vi "MP_Conver_HumanToMachine.vi"(6 "Vel_In (ft/s)":dbl, 7 "Pos_In (ft)":dbl, 8 "CPR":dbl, 9 "Diameter (ft)":dbl) -> (2 "Vel_Out (u/100ms)":dbl, 3 "Pos_Out (u)":dbl)   [LabVIEW 2017]
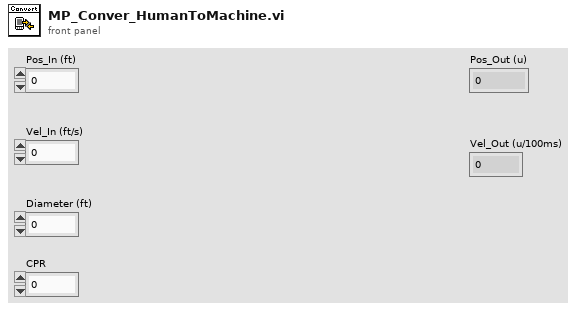
[diagram p1: front panel]
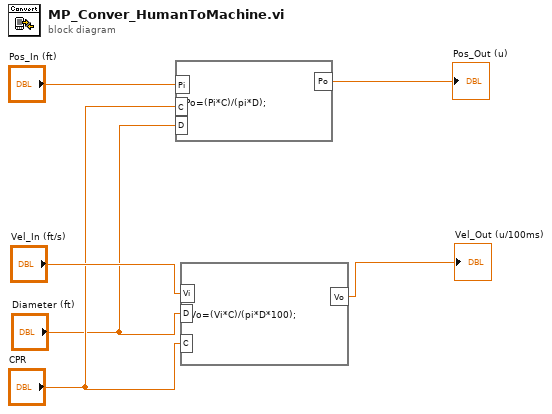
[diagram p0: block diagram]
diagram:
  n1 = formula code="Po=(Pi*C)/(pi*D);"("Pi"="Pos_In (ft)", "C"="CPR", "D"="Diameter (ft)") -> ("Po"=→"Pos_Out (u)":dbl)
  n2 = formula code="Vo=(Vi*C)/(pi*D*100);"("Vi"="Vel_In (ft/s)", "D"="Diameter (ft)", "C"="CPR") -> ("Vo"=→"Vel_Out (u/100ms)":dbl)
